vi "Initialize.vi"(8 "error in":errorcluster, 11 "Plugin in":refnum<class "AutomotiveDataSimulator.lvclass">) -> (0 "error out":errorcluster, 3 "Plugin out":refnum<class "AutomotiveDataSimulator.lvclass">)   [LabVIEW 2020, in "AutomotiveDataSimulator.lvlib" / "AutomotiveDataSimulator.lvclass"]
uses:
  AutomotiveDataSimulator.lvclass
  C:/Program Files/National Instruments/LabVIEW 2020/vi.lib/FlexLogger/SDK/PluginSDK.lvlibp/PEFClasses/SDK/Plugin/Plugin.lvclass
  <vilib>/FlexLogger/SDK/PluginSDK.lvlibp/PEFClasses/SDK/System Interface/Resampling Mode.ctl
  <vilib>/FlexLogger/SDK/PluginSDK.lvlibp/PEFClasses/SDK/Producer Channel/Producer Channel.lvclass
  C:/Program Files/National Instruments/LabVIEW 2020/vi.lib/FlexLogger/SDK/PluginSDK.lvlibp/PEFClasses/SDK/Channel/Channel.lvclass
  <vilib>/FlexLogger/SDK/PluginSDK.lvlibp/PEFClasses/SDK/Plugin/ParameterAccess/Write N Channel.vi
  <vilib>/FlexLogger/SDK/PluginSDK.lvlibp/PEFClasses/SDK/Plugin/ParameterAccess/Write Enum.vi
  <vilib>/FlexLogger/SDK/PluginSDK.lvlibp/PEFClasses/SDK/Derived Timing Producer Channel/Create Derived Time Producer Channel.vi
  <vilib>/FlexLogger/SDK/PluginSDK.lvlibp/PEFClasses/SDK/Plugin/Plugin.lvclass
  <vilib>/FlexLogger/SDK/PluginSDK.lvlibp
  <vilib>/FlexLogger/SDK/PluginSDK.lvlibp/PEFClasses/SDK/System Interface/System Interface.lvclass
  <vilib>/FlexLogger/SDK/PluginSDK.lvlibp/PEFClasses/SDK/Derived Timing Producer Channel/Derived Timing Producer Channel.lvclass
  C:/Program Files/National Instruments/LabVIEW 2020/vi.lib/FlexLogger/SDK/PluginSDK.lvlibp/PEFClasses/SDK/Processing Element/Processing Element.lvclass
  C:/Users/dgrajale/Desktop/Flexlogger Project/Flexlogger Plugins/AutomotiveDataSimulator/AutomotiveDataSimulator.lvclass
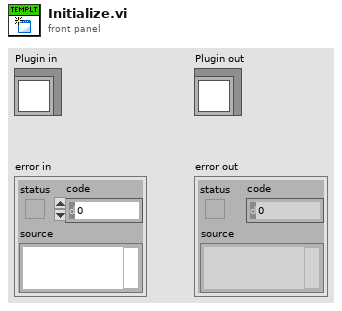
[diagram p1: front panel]
types:
  T1 = typedef "PluginSDK.lvlibp/System Interface.lvclass/Resampling Mode.ctl" = enum16{"No Resampling", "Custom Rate", "Maximum Rate", "Minimum Rate"}
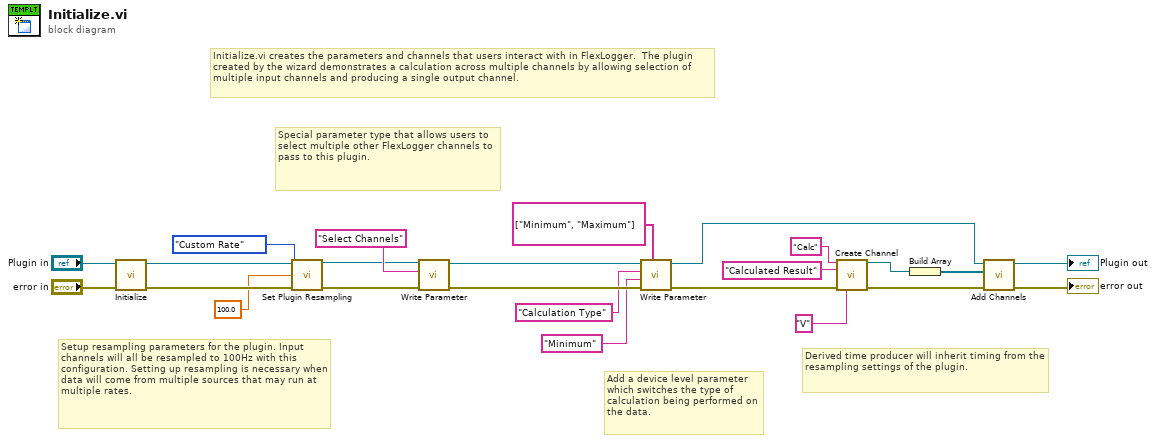
[diagram p0: block diagram]
diagram:
  # "Add a device level parameter which switches the type of calculation being performed on the data."
  # "Setup resampling parameters for the plugin. Input channels will all be resampled to 100Hz with this configuration. Setting up resampling is necessary when data will come from multiple sources that may run at multiple rates."
  # "Derived time producer will inherit timing from the resampling settings of the plugin."
  # "Special parameter type that allows users to select multiple other FlexLogger channels to pass to this plugin."
  # "Initialize.vi creates the parameters and channels that users interact with in FlexLogger.  The plugin created by the wizard demonstrates a calculation across multiple channels by allowing selection of multiple input channels and producing a single output channel."
  n1 = call-parent "Initialize.vi"("error in (no error)"="error in", "Plugin in"="Plugin in") -> ("error out"=w19:errorcluster, "Plugin out"=w20:refnum<class "AutomotiveDataSimulator.lvclass">)  [unwired: 8 in]
  n2 = call <vilib>:"Set Plugin Resampling.vi"("Plugin in"=w20, "Resampling Mode"=Resampling_Mode."Custom Rate", "Resampling Rate (Hz)"=100.0, "error in (no error)"=w19) -> ("Plugin out"=w18:refnum<class "AutomotiveDataSimulator.lvclass">, "error out"=w17:errorcluster)  [unwired: 10 in]
  n3 = call-poly <vilib>:"Write Parameter.vi"("error in (no error)"=w17, "Name (Unique Channel Identifier)"="Select Channels" ("Name"), "Plugin in"=w18) -> ("error out"=w9:errorcluster, "Plugin out"=w10:refnum<class "AutomotiveDataSimulator.lvclass">)  [unwired: 7 in]
  n4 = call-poly <vilib>:"Write Parameter.vi"("Possible Values"=string[] ["Minimum", "Maximum"], "error in (no error)"=w9, "Current Value"="Minimum", "Name"="Calculation Type", "Plugin in"=w10) -> ("error out"=w7:errorcluster, "Plugin out"=w8:refnum<class "AutomotiveDataSimulator.lvclass">)  [unwired: 5 in]
  n5 = call-poly <vilib>:"Create Channel.vi"("Unique Channel Identifier"="Calc", "Default Channel Name"="Calculated Result" ("Unique Channel Identifier"), "error in (no error)"=w7, "Unit"="V") -> ("Producer Channel"=w15:refnum<class "Producer Channel.lvclass">, "error out"=w13:errorcluster)  [unwired: 10 in]
  n6 = Build Array(w15) -> (w14:refnum<class "Producer Channel.lvclass">[])
  n7 = call <vilib>:"Add Channels.vi"("error in (no error)"=w13, "Channels"=w14, "Plugin in"=w8) -> ("error out"=→"error out":errorcluster, "Plugin out"=→"Plugin out":refnum<class "AutomotiveDataSimulator.lvclass">)  [unwired: 7 in]
